vi "Lyapunov Equations.vi"   [LabVIEW 2012, in "NI_AALPro.lvlib"]
doc: "Solves the Lyapunov matrix equation. The data types you wire to the <B>A</B> and <B>B</B> inputs determine the polymorphic instance to use."
uses:
  NI_AALPro.lvlib
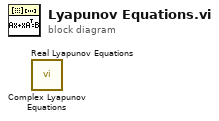
[diagram p0: block diagram]
diagram:
  n1 = call "Complex Lyapunov Equations.vi"() -> ()  [unwired: 9 in, 3 out]
  n2 = call "Real Lyapunov Equations.vi"() -> ()  [unwired: 9 in, 3 out]
